vi "pmu_Get Reporting Raw Data.vi"(0 "magnitudes [RMS]":dbl[][](array[numeric]), 1 "buffer length":i32=10, 2 "reset? (F)":bool, 5 "phases [pi]":dbl[][](array[numeric]), 7 "timestamps out":dbl[][](array[numeric]), 9 "buffered GPS information":T1[](array[typedef]), 11 "max t0 index":i32, 12 "reporting rate":i16, 13 "min final timestamp":timestamp, 14 "current reporting time":timestamp) -> (4 "reporting raw data":T2, 6 "reporting GPS information":T1)   [LabVIEW 2013, in "NI_EP_PMU.lvlib"]
uses:
  <vilib>/addons/Electrical Power/PMU/NI_EP_PMU.lvlib
  <vilib>/addons/Electrical Power/PMU/Common/Controls/pmu_GPS Info.ctl
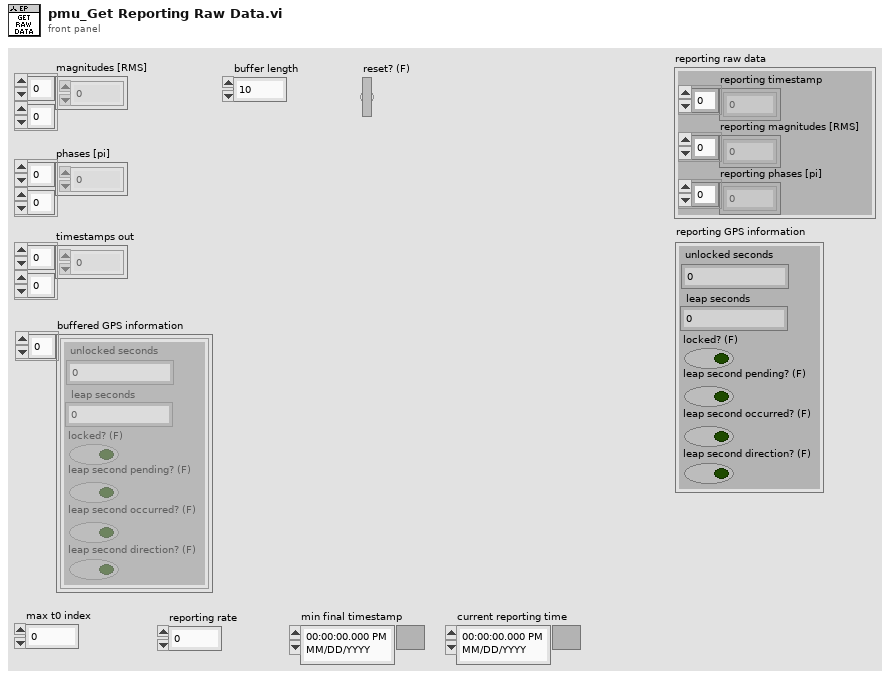
[diagram p1: front panel]
types:
  T1 = typedef "NI_EP_PMU.lvlib/pmu_GPS Info.ctl" = cluster{"unlocked seconds":u32, "leap seconds":i8, "locked? (F)":bool, "leap second pending? (F)":bool, "leap second occurred? (F)":bool, "leap second direction? (F)":bool}
  T2 = cluster{"reporting timestamp":dbl[], "reporting magnitudes [RMS]":dbl[], "reporting phases [pi]":dbl[]}
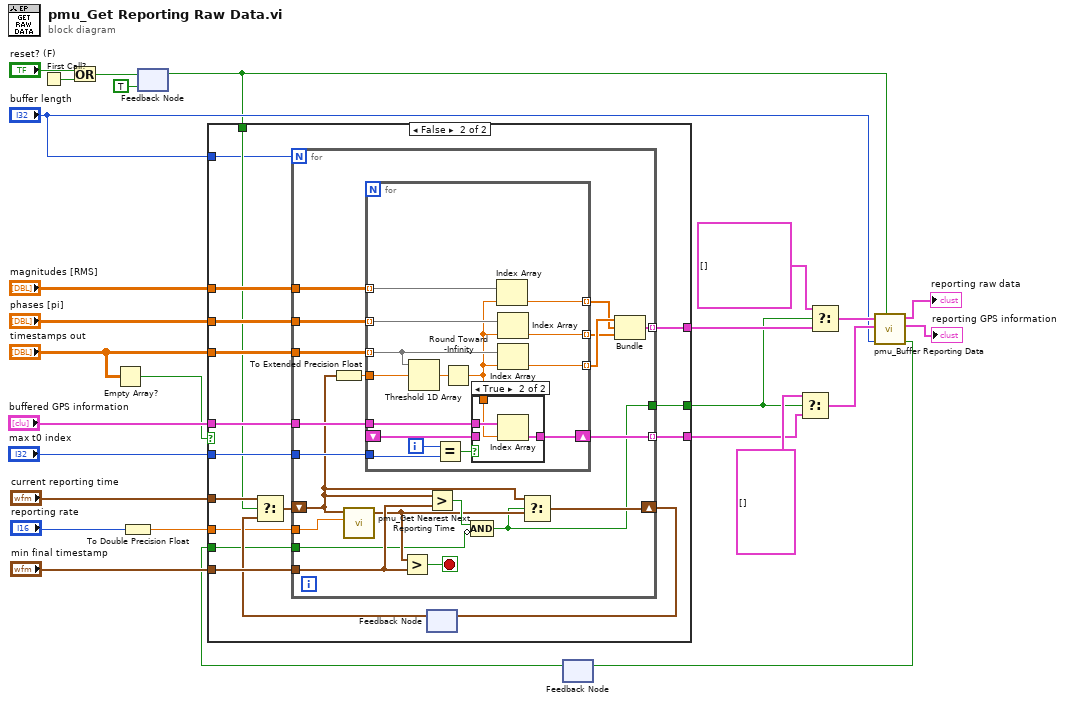
[diagram p0: block diagram]
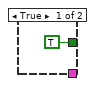
[diagram p2: hidden frame]
diagram:
  n1 = First Call?() -> (First Call?: T/F=w20:bool)
  n2 = Or(x="reset? (F)", y=w20) -> (x .or. y?=w18:bool)
  n3 = Empty Array?(array="timestamps out") -> (empty?=w10:bool)
  n4 = To Double Precision Float(number="reporting rate") -> (double precision float=w1:dbl)
  n5 = feedback #1(TRUE) -> (w4:bool)
  n6 = feedback-in #1(w18) -> ()
  n7 = feedback #2() -> (w3:bool)  [unwired: 1 in]
  n8 = case shown="False" w10 {
    tunnel: "max t0 index" -> [_ w45]
    tunnel: "buffered GPS information" -> [_ w44]
    tunnel: "phases [pi]" -> [_ w43]
    tunnel: "magnitudes [RMS]" -> [_ w42]
    tunnel: "timestamps out" -> [_ w41]
    tunnel: w1 -> [_ w30]
    tunnel: "min final timestamp" -> [_ w40]
    tunnel: "current reporting time" -> [_ w38]
    tunnel: w4 -> [_ w36]
    tunnel: "buffer length" -> [_ w35]
    tunnel: [_ w33] -> w17
    tunnel: [TRUE w32] -> w6
    tunnel: [_ w31] -> w13
    tunnel: w3 -> [_ w29]
    frame True {
    }
    frame False {
      n9 = feedback #3() -> (w34:timestamp)  [unwired: 1 in]
      n10 = Select(t=w38, s=w36, f=w34) -> (s? t:f=w39:timestamp)
      n11 = for {
        N: w35 -> [_]
        tunnel: w42 -> [w65]
        tunnel: w43 -> [w64]
        tunnel: w41 -> [w63]
        tunnel: [w61] -> w33 mode=indexing
        tunnel: w45 -> [w60]
        tunnel: w44 -> [w59]
        tunnel: [w58] -> w31 mode=indexing
        tunnel: w40 -> [w56]
        shift-right: [w55] -> w37
        shift-left: w39 -> [w48]
        tunnel: [w47] -> w32
        tunnel: w30 -> [w49]
        tunnel: w29 -> [w46]
        stop <- w57 stop-if-true
        n12 = To Extended Precision Float(1:w48) -> (0:w51:ext)
        n13 = call <vilib>:"pmu_Get Nearest Next Reporting Time.vi"("reporting rate"=w49, "time in"=w48) -> ("reporting time"=w50:timestamp)  [unwired: 8 in, 1 out]
        n14 = for {
          tunnel: w63 -> [w71] mode=indexing
          tunnel: w51 -> [w79]
          tunnel: w65 -> [w68] mode=indexing
          tunnel: w64 -> [w70] mode=indexing
          tunnel: [w78] -> w62 mode=indexing
          tunnel: w60 -> [w76]
          tunnel: w59 -> [w74]
          shift-right: [w73] -> w58
          shift-left: _ -> [w72]
          tunnel: [w69] -> w53 mode=indexing
          tunnel: [w66] -> w52 mode=indexing
          i -> [w77]
          n15 = Threshold 1D Array(2:w79, 3:w71) -> (0:w80:dbl)  [unwired: 1 in]
          n16 = Equal?(x=w77, y=w76) -> (x = y?=w75:bool)
          n17 = Round Toward -Infinity(1:w80) -> (0:w67:dbl)
          n18 = case shown="True" w75 {
            tunnel: w74 -> [_ w84]
            tunnel: w67 -> [_ w83]
            tunnel: [w81 w82] -> w73
            tunnel: w72 -> [w81 _]
            frame False {
            }
            frame True {
              n19 = Index Array(array=w84, index=w83) -> (element=w82:T1)
            }
          }
          n20 = Index Array(array=w68, index=w67) -> (element=w66:dbl)
          n21 = Index Array(array=w70, index=w67) -> (element=w69:dbl)
          n22 = Index Array(array=w71, index=w67) -> (element=w78:dbl)
        }
        n23 = Greater?(x=w50, y=w56) -> (0:w57:bool)
        n24 = Greater?(x=w48, y=w56) -> (0:w54:bool)
        n25 = Compound Arithmetic op=AND(w54, invert w46) -> (w47:bool)
        n26 = Select(t=w48, s=w47, f=w50) -> (s? t:f=w55:timestamp)
        n27 = Bundle(w62, w52, w53) -> (w61:cluster{dbl[], dbl[], dbl[]})  [unwired: 1 in]
      }
      n28 = feedback-in #3(w37) -> ()
    }
  }
  n29 = Select(t=T1[] [], s=w6, f=w13) -> (s? t:f=w12:T1[])
  n30 = Select(t=cluster{dbl[], dbl[], dbl[]}[] [], s=w6, f=w17) -> (s? t:f=w15:cluster{dbl[], dbl[], dbl[]}[])
  n31 = call <vilib>:"pmu_Buffer Reporting Data.vi"("reset? (F)"=w4, "buffer length"="buffer length", "GPS information"=w12, "raw data"=w15) -> ("empty?"=w2:bool, "reporting GPS information"=→"reporting GPS information":T1, "reporting raw data"=→"reporting raw data":T2)  [unwired: 5 in]
  n32 = feedback-in #2(w2) -> ()
